vi "2_3.vi"() -> ()   [LabVIEW 2017]
panel:
  in  "P Sensor Max Output":i8
  in  "P Sensor Min Output":i8
  in  "Max Measure Range":i16
  in  "Min Measure Range":i8
  out "Pressure Guage [Bar]":dbl
  out "Bar/V":dbl
  out "Pressure [Bar]":dbl(knob) scale=0.0..10.0
  in  "Cluster 2":cluster{"Cuurent Sensor Output [V]":dbl} {"Cuurent Sensor Output [V]" scale=0.0..5.0}
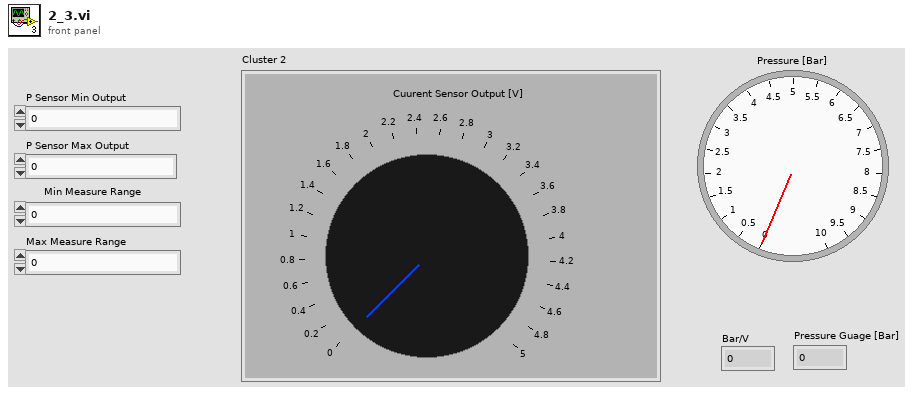
[diagram p1: front panel]
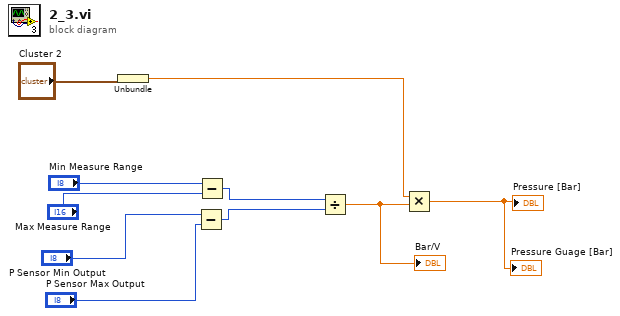
[diagram p0: block diagram]
diagram:
  n1 = Unbundle("Cluster 2") -> ("Cuurent Sensor Output [V]"=w7:dbl)
  n2 = Subtract(x="P Sensor Min Output", y="P Sensor Max Output") -> (x-y=w9:i8)
  n3 = Subtract(x="Min Measure Range", y="Max Measure Range") -> (x-y=w10:i16)
  n4 = Divide(x=w10, y=w9) -> (x/y=w6:dbl)
  "Bar/V" <- w6
  n5 = Multiply(x=w7, y=w6) -> (x*y=→"Pressure [Bar]" →"Pressure Guage [Bar]":dbl)
